vi "HandleTab.vi"(6 "Forward?":bool=TRUE, 8 "error in (no error)":errorcluster, 11 "TabbedControls":T1[](array[typedef])) -> (0 "error out":errorcluster, 3 "Discard?":bool)   [LabVIEW 2020, in "ContextHelpEditor.lvlib"]
uses:
  ContextHelpEditor.lvlib
  TabbedControl--cluster.ctl
  TabChange State--cluster.ctl
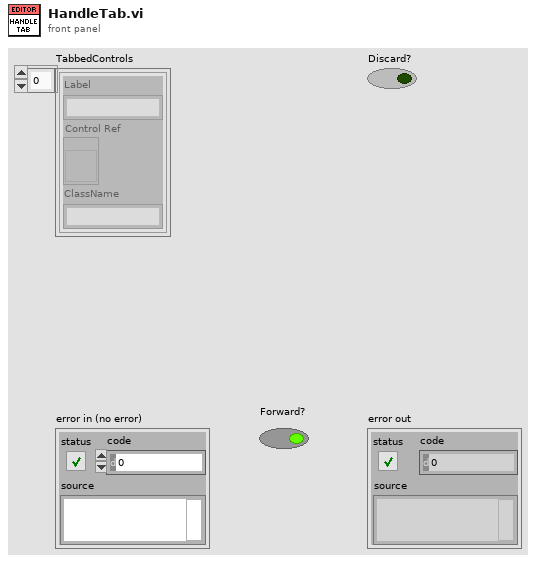
[diagram p1: front panel]
types:
  T1 = typedef "ContextHelpEditor.lvlib/TabbedControl--cluster.ctl" = cluster{"Label":string, "Control Ref":refnum<vi>, "ClassName":string}
  T2 = typedef "ContextHelpEditor.lvlib/TabChange State--cluster.ctl" = enum16{"CHECK_CURRENT_TYPE", "CHECK_PREVIOUS_TYPE", "CHECK_NEXT_TYPE", "CHECK_JUMP_INNER_MCLISTBOX", "JUMP_CURRENT_FW_MCLISTBOX", "JUMP_CURRENT_BACK_MCLISTBOX", "ACTIVATE_FIRST_ELEM_MCLISTBOX", "ACTIVATE_LAST_ELEM_MCLISTBOX", "ACTIVATE_NEXT_CONTROL", "ACTIVATE_PREV_CONTROL"}
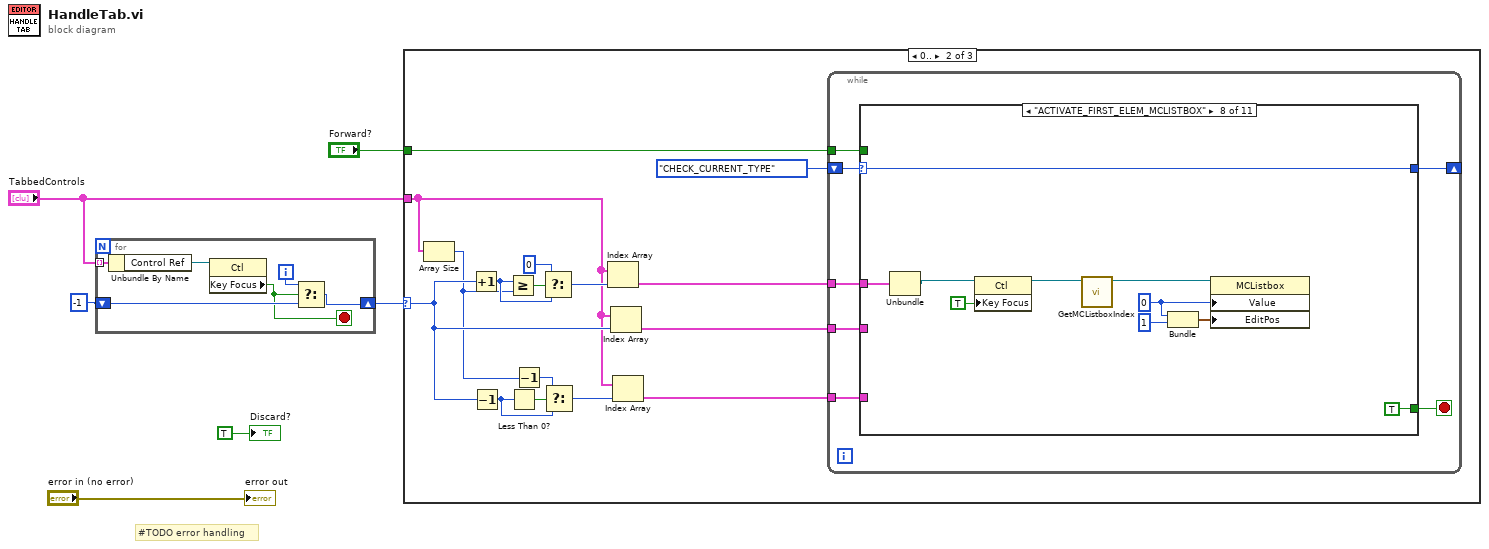
[diagram p0: block diagram]
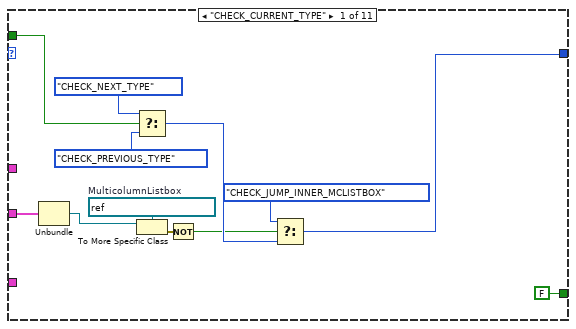
[diagram p3: hidden frame]
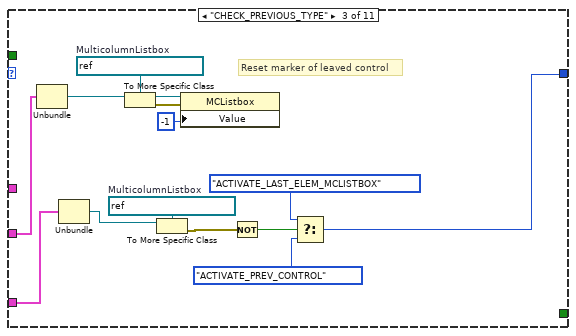
[diagram p5: hidden frame]
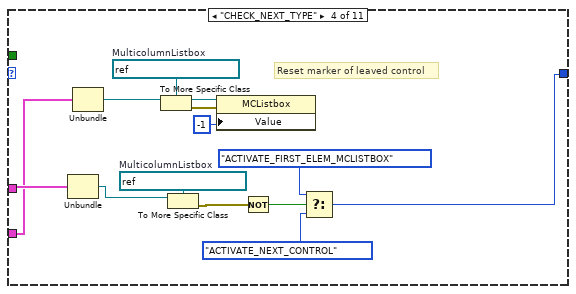
[diagram p6: hidden frame]
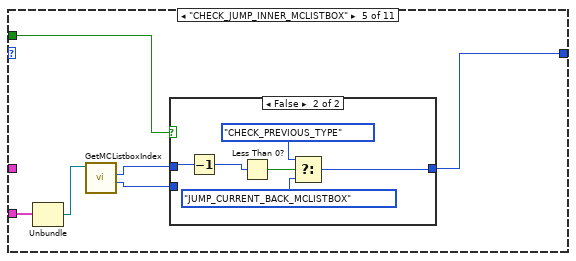
[diagram p7: hidden frame]
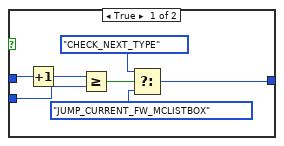
[diagram p8: hidden frame]
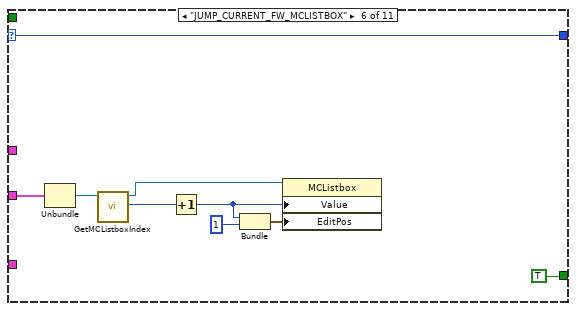
[diagram p9: hidden frame]
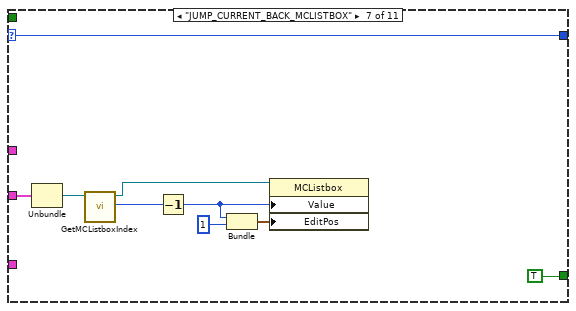
[diagram p10: hidden frame]
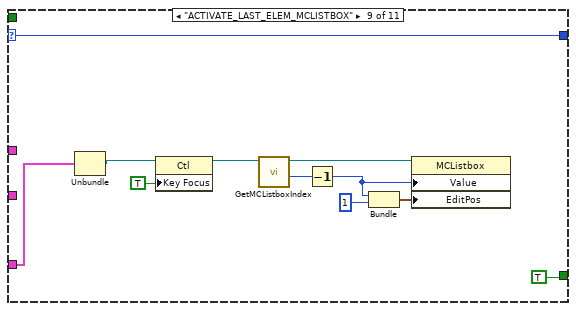
[diagram p11: hidden frame]
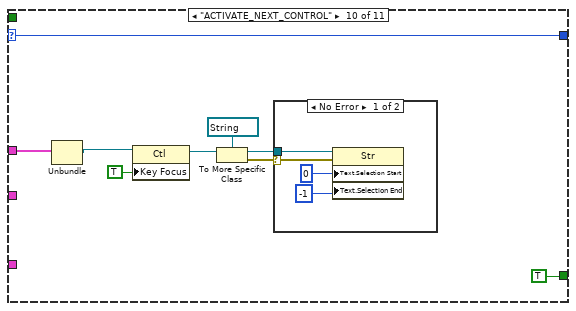
[diagram p12: hidden frame]
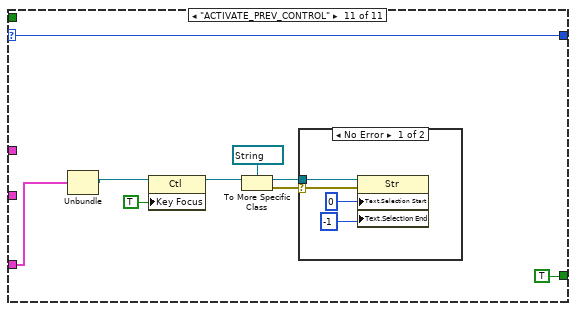
[diagram p14: hidden frame]
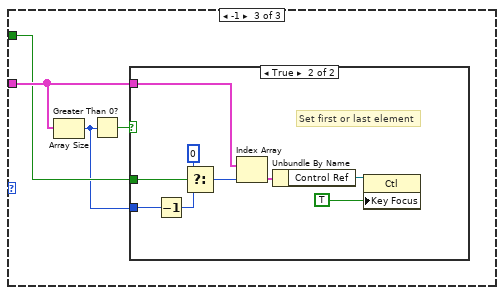
[diagram p16: hidden frame]
diagram:
  # "#TODO error handling"
  n1 = for {
    tunnel: "TabbedControls" -> [w12] mode=indexing
    shift-right: [w10] -> w3
    shift-left: -1 -> [w8]
    i -> [w9]
    stop <- w7 stop-if-true
    n2 = Unbundle By Name(w12) -> ("Control Ref"=w11:refnum<vi>)
    n3 = property class="Ctl"(reference=w11) -> ("Key Focus"=w7:bool)  [unwired: 1 in, 2 out]
    n4 = Select(t=w9, s=w7, f=w8) -> (s? t:f=w10:i32)
  }
  n5 = case shown="0.." w3 {
    selector: w3 -> [_ w23 _]
    tunnel: "TabbedControls" -> [_ w19 w164]
    tunnel: "Forward?" -> [_ w16 w162]
    frame Default {
    }
    frame 0.. {
      n6 = Array Size(array=w19) -> (size(s)=w21:i32)
      n7 = Increment(x=w23) -> (x+1=w25:i32)
      n8 = Decrement(x=w23) -> (x-1=w22:i32)
      n9 = Greater Or Equal?(x=w25, y=w21) -> (x >= y?=w28:bool)
      n10 = Less Than 0?(x=w22) -> (x < 0?=w24:bool)
      n11 = Decrement(x=w21) -> (x-1=w20:i32)
      n12 = Select(t=0, s=w28, f=w25) -> (s? t:f=w26:i32)
      n13 = Select(t=w20, s=w24, f=w22) -> (s? t:f=w18:i32)
      n14 = Index Array(array=w19, index=w26) -> (element=w15:T1)
      n15 = Index Array(array=w19, index=w23) -> (element=w14:T1)
      n16 = Index Array(array=w19, index=w18) -> (element=w13:T1)
      n17 = while {
        shift-right: [w34] -> _
        shift-left: TabChange_State--cluster."CHECK_CURRENT_TYPE" -> [w35]
        tunnel: w16 -> [w33]
        tunnel: w15 -> [w31]
        tunnel: w14 -> [w30]
        tunnel: w13 -> [w29]
        stop <- w32 stop-if-true
        n18 = case shown="\"ACTIVATE_FIRST_ELEM_MCLISTBOX\"" w35 {
          selector: w35 -> [_ w48 _ _ _ w96 w105 w116 w124 w139 w152]
          tunnel: [w41 w48 w59 w73 w79 w96 w105 w116 w124 w139 w152] -> w34
          tunnel: w33 -> [w45 _ _ _ w80 _ _ _ _ _ _]
          tunnel: [FALSE _ _ _ _ TRUE TRUE TRUE TRUE TRUE TRUE] -> w32
          tunnel: w31 -> [_ _ _ w76 _ _ _ w120 _ w141 _]
          tunnel: w30 -> [w46 _ w56 w67 w82 w103 w107 _ _ _ _]
          tunnel: w29 -> [_ _ w60 _ _ _ _ _ w130 _ w154]
          frame "CHECK_CURRENT_TYPE" {
            w39 = refnum<vi> refnum  # MulticolumnListbox
            n19 = Unbundle(w46) -> ("Control Ref"=w36:refnum<vi>)  [unwired: 2 out]
            n20 = Select(t=TabChange_State--cluster."CHECK_NEXT_TYPE", s=w45, f=TabChange_State--cluster."CHECK_PREVIOUS_TYPE") -> (s? t:f=w42:T2)
            n21 = To More Specific Class(target class=w39, reference=w36) -> (error out=w38:errorcluster)  [unwired: 1 in, 1 out]
            n22 = Not(x=w38) -> (.not. x?=w37:bool)
            n23 = Select(t=TabChange_State--cluster."CHECK_JUMP_INNER_MCLISTBOX", s=w37, f=w42) -> (s? t:f=w41:T2)
          }
          frame Default {
          }
          frame "CHECK_PREVIOUS_TYPE" {
            w52 = refnum<vi> refnum  # MulticolumnListbox
            w53 = refnum<vi> refnum  # MulticolumnListbox
            # "Reset marker of leaved control"
            n24 = Unbundle(w56) -> ("Control Ref"=w57:refnum<vi>)  [unwired: 2 out]
            n25 = Unbundle(w60) -> ("Control Ref"=w49:refnum<vi>)  [unwired: 2 out]
            n26 = To More Specific Class(target class=w53, reference=w57) -> (specific class reference=w54:refnum<vi>, error out=w55:errorcluster)  [unwired: 1 in]
            n27 = To More Specific Class(target class=w52, reference=w49) -> (error out=w51:errorcluster)  [unwired: 1 in, 1 out]
            n28 = property class="MCListbox"(reference=w54, error in=w55, "Value"=-1) -> ()  [unwired: 2 out]
            n29 = Not(x=w51) -> (.not. x?=w50:bool)
            n30 = Select(t=TabChange_State--cluster."ACTIVATE_LAST_ELEM_MCLISTBOX", s=w50, f=TabChange_State--cluster."ACTIVATE_PREV_CONTROL") -> (s? t:f=w59:T2)
          }
          frame "CHECK_NEXT_TYPE" {
            w66 = refnum<vi> refnum  # MulticolumnListbox
            w68 = refnum<vi> refnum  # MulticolumnListbox
            # "Reset marker of leaved control"
            n31 = Unbundle(w76) -> ("Control Ref"=w65:refnum<vi>)  [unwired: 2 out]
            n32 = Unbundle(w67) -> ("Control Ref"=w71:refnum<vi>)  [unwired: 2 out]
            n33 = To More Specific Class(target class=w68, reference=w71) -> (specific class reference=w69:refnum<vi>, error out=w70:errorcluster)  [unwired: 1 in]
            n34 = To More Specific Class(target class=w66, reference=w65) -> (error out=w64:errorcluster)  [unwired: 1 in, 1 out]
            n35 = property class="MCListbox"(reference=w69, error in=w70, "Value"=-1) -> ()  [unwired: 2 out]
            n36 = Not(x=w64) -> (.not. x?=w63:bool)
            n37 = Select(t=TabChange_State--cluster."ACTIVATE_FIRST_ELEM_MCLISTBOX", s=w63, f=TabChange_State--cluster."ACTIVATE_NEXT_CONTROL") -> (s? t:f=w73:T2)
          }
          frame "CHECK_JUMP_INNER_MCLISTBOX" {
            n38 = Unbundle(w82) -> ("Control Ref"=w81:refnum<vi>)  [unwired: 2 out]
            n39 = call "GetMCListboxIndex.vi"("Control in"=w81) -> ("Size"=w78:i32, "Index"=w77:i32)  [unwired: 7 in, 2 out]
            n40 = case shown="False" w80 {
              tunnel: w78 -> [w87 _]
              tunnel: w77 -> [w86 w94]
              tunnel: [w84 w91] -> w79
              frame True {
                n41 = Increment(x=w86) -> (x+1=w89:i32)
                n42 = Greater Or Equal?(x=w89, y=w87) -> (x >= y?=w88:bool)
                n43 = Select(t=TabChange_State--cluster."CHECK_NEXT_TYPE", s=w88, f=TabChange_State--cluster."JUMP_CURRENT_FW_MCLISTBOX") -> (s? t:f=w84:T2)
              }
              frame False {
                n44 = Decrement(x=w94) -> (x-1=w92:i32)
                n45 = Less Than 0?(x=w92) -> (x < 0?=w95:bool)
                n46 = Select(t=TabChange_State--cluster."CHECK_PREVIOUS_TYPE", s=w95, f=TabChange_State--cluster."JUMP_CURRENT_BACK_MCLISTBOX") -> (s? t:f=w91:T2)
              }
            }
          }
          frame "JUMP_CURRENT_FW_MCLISTBOX" {
            n47 = Unbundle(w103) -> ("Control Ref"=w104:refnum<vi>)  [unwired: 2 out]
            n48 = call "GetMCListboxIndex.vi"("Control in"=w104) -> ("Index"=w102:i32, "MCListbox out"=w98:refnum<vi>)  [unwired: 7 in, 2 out]
            n49 = Increment(x=w102) -> (x+1=w99:i32)
            n50 = Bundle(w99, "index"=1) -> (w100:cluster{i32, "index":i32})  [unwired: 1 in]
            n51 = property class="MCListbox"(reference=w98, "Value"=w99, "EditPos"=w100) -> ()  [unwired: 1 in, 2 out]
          }
          frame "JUMP_CURRENT_BACK_MCLISTBOX" {
            n52 = Unbundle(w107) -> ("Control Ref"=w113:refnum<vi>)  [unwired: 2 out]
            n53 = call "GetMCListboxIndex.vi"("Control in"=w113) -> ("Index"=w112:i32, "MCListbox out"=w108:refnum<vi>)  [unwired: 7 in, 2 out]
            n54 = Decrement(x=w112) -> (x-1=w109:i32)
            n55 = Bundle(w109, "index"=1) -> (w110:cluster{i32, "index":i32})  [unwired: 1 in]
            n56 = property class="MCListbox"(reference=w108, "Value"=w109, "EditPos"=w110) -> ()  [unwired: 1 in, 2 out]
          }
          frame "ACTIVATE_FIRST_ELEM_MCLISTBOX" {
            w118 = 0 ("index")
            n57 = Unbundle(w120) -> ("Control Ref"=w119:refnum<vi>)  [unwired: 2 out]
            n58 = property class="Ctl"(reference=w119, "Key Focus"=TRUE) -> (reference out=w115:refnum<vi>)  [unwired: 1 in, 1 out]
            n59 = call "GetMCListboxIndex.vi"("Control in"=w115) -> ("MCListbox out"=w121:refnum<vi>)  [unwired: 7 in, 3 out]
            n60 = Bundle("index"=w118, "index"=1) -> (w122:cluster{"index":i32, "index":i32})  [unwired: 1 in]
            n61 = property class="MCListbox"(reference=w121, "Value"=w118, "EditPos"=w122) -> ()  [unwired: 1 in, 2 out]
          }
          frame "ACTIVATE_LAST_ELEM_MCLISTBOX" {
            n62 = Unbundle(w130) -> ("Control Ref"=w131:refnum<vi>)  [unwired: 2 out]
            n63 = property class="Ctl"(reference=w131, "Key Focus"=TRUE) -> (reference out=w126:refnum<vi>)  [unwired: 1 in, 1 out]
            n64 = call "GetMCListboxIndex.vi"("Control in"=w126) -> ("Size"=w128:i32, "MCListbox out"=w132:refnum<vi>)  [unwired: 7 in, 2 out]
            n65 = Decrement(x=w128) -> (x-1=w129:i32)
            n66 = Bundle(w129, "index"=1) -> (w133:cluster{i32, "index":i32})  [unwired: 1 in]
            n67 = property class="MCListbox"(reference=w132, "Value"=w129, "EditPos"=w133) -> ()  [unwired: 1 in, 2 out]
          }
          frame "ACTIVATE_NEXT_CONTROL" {
            n68 = Unbundle(w141) -> ("Control Ref"=w143:refnum<vi>)  [unwired: 2 out]
            n69 = property class="Ctl"(reference=w143, "Key Focus"=TRUE) -> (reference out=w138:refnum<vi>)  [unwired: 1 in, 1 out]
            n70 = To More Specific Class(target class=refnum<vi> refnum ("VI Title"), reference=w138) -> (specific class reference=w137:refnum<vi>, error out=w135:errorcluster)  [unwired: 1 in]
            n71 = case shown="No Error" w135 {
              selector: w135 -> [w144 _]
              tunnel: w137 -> [w147 _]
              frame No Error {
                n72 = property class="Str"(reference=w147, error in=w144, "Text.Selection Start"=u32 0 ("Text.Selection:Start"), "Text.Selection End"=-1 ("Text.Selection:Start")) -> ()  [unwired: 2 out]
              }
              frame Error {
              }
            }
          }
          frame "ACTIVATE_PREV_CONTROL" {
            n73 = Unbundle(w154) -> ("Control Ref"=w156:refnum<vi>)  [unwired: 2 out]
            n74 = property class="Ctl"(reference=w156, "Key Focus"=TRUE) -> (reference out=w148:refnum<vi>)  [unwired: 1 in, 1 out]
            n75 = To More Specific Class(target class=refnum<vi> refnum ("VI Title"), reference=w148) -> (specific class reference=w151:refnum<vi>, error out=w149:errorcluster)  [unwired: 1 in]
            n76 = case shown="No Error" w149 {
              selector: w149 -> [w157 _]
              tunnel: w151 -> [w160 _]
              frame No Error {
                n77 = property class="Str"(reference=w160, error in=w157, "Text.Selection Start"=u32 0 ("Text.Selection:Start"), "Text.Selection End"=-1 ("Text.Selection:Start")) -> ()  [unwired: 2 out]
              }
              frame Error {
              }
            }
          }
        }
      }
    }
    frame -1 {
      n78 = Array Size(array=w164) -> (size(s)=w161:i32)
      n79 = Greater Than 0?(x=w161) -> (x > 0?=w163:bool)
      n80 = case shown="True" w163 {
        tunnel: w164 -> [_ w172]
        tunnel: w162 -> [_ w169]
        tunnel: w161 -> [_ w165]
        frame False {
        }
        frame True {
          # "Set first or last element"
          n81 = Decrement(x=w165) -> (x-1=w166:i32)
          n82 = Select(t=0, s=w169, f=w166) -> (s? t:f=w167:i32)
          n83 = Index Array(array=w172, index=w167) -> (element=w171:T1)
          n84 = Unbundle By Name(w171) -> ("Control Ref"=w170:refnum<vi>)
          n85 = property class="Ctl"(reference=w170, "Key Focus"=TRUE) -> ()  [unwired: 1 in, 2 out]
        }
      }
    }
  }
  "Discard?" <- TRUE
  "error out" <- "error in (no error)"
